vi "Finish.vi"   [LabVIEW 2013]
doc: "This VI is called just before exiting. It is expected to close I/O refnum, save collected data, etc."
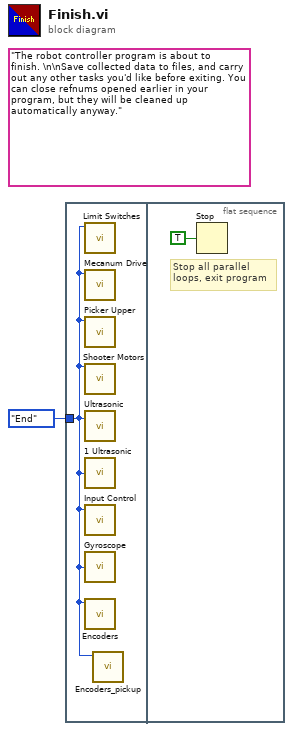
[diagram p0: block diagram]
diagram:
  (unwired) "The robot controller program is about to finish. \n\nSave collected data to files, and carry out any other tasks you'd like before exiting. You can close refnums opened earlier in your program, but they will be cleaned up automatically anyway."
  n1 = flat-sequence {
    tunnel: enum16{"Open", "Run", "End"}."End" ("State Control") -> [w2]
    frame #0 {
      n2 = call "Limit Switches.vi"("State Control"=w2) -> ()  [unwired: 7 in, 4 out]
      n3 = call "Mecanum Drive.vi"("State Control"=w2) -> ()  [unwired: 7 in]
      n4 = call "Picker Upper.vi"("State Control"=w2) -> ()  [unwired: 10 in, 1 out]
      n5 = call "Shooter Motors.vi"("State Control"=w2) -> ()  [unwired: 16 in, 3 out]
      n6 = call "Ultrasonic.vi"("State Control"=w2) -> ()  [unwired: 2 in]
      n7 = call "1 Ultrasonic.vi"("State Control"=w2) -> ()  [unwired: 1 out]
      n8 = call "Input Control.vi"("State"=w2) -> ()  [unwired: 2 in, 3 out]
      n9 = call "Gyroscope.vi"("State Control"=w2) -> ()  [unwired: 2 out]
      n10 = call "Encoders.vi"("State Control"=w2) -> ()  [unwired: 3 in, 4 out]
      n11 = call "Encoders_pickup.vi"("State Control"=w2) -> ()  [unwired: 3 in, 4 out]
    }
    frame #1 {
      # "Stop all parallel\nloops, exit program"
      n12 = Stop(stop? (T)=TRUE ("Quit")) -> ()
    }
  }
